vi "Laucher.vi"() -> ()   [LabVIEW 2015]
uses:
  <vilib>/ActorFramework/Actor/Actor.lvclass
panel:
  in  "硬件查询数据间隔":u32=10
  in  "硬件端口":refnum<visa-resource-name>="COM30"
  in  "服务器查询数据间隔":i32=10
  in  "服务器端口":refnum<visa-resource-name>="COM29"
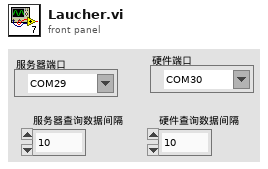
[diagram p1: front panel]
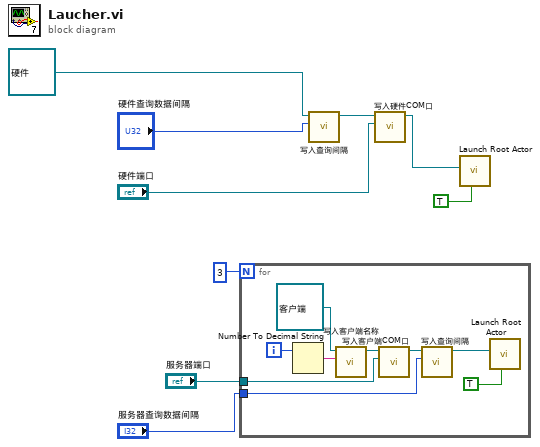
[diagram p0: block diagram]
diagram:
  n1 = for {
    N: 3 -> [_]
    tunnel: "服务器端口" -> [w13]
    tunnel: "服务器查询数据间隔" -> [w12]
    i -> [w17]
    n2 = Number To Decimal String(number=w17) -> (decimal integer string=w16:string)  [unwired: 1 in]
    n3 = call-dynamic "写入客户端名称.vi"("客户端名称"=w16, "客户端输入"=refnum<class "客户端.lvclass"> refnum ("客户端.lvlib:客户端.lvclass")) -> ("客户端输出"=w14:refnum<class "客户端.lvclass">)  [unwired: 8 in, 1 out]
    n4 = call-dynamic "写入客户端COM口.vi"("客户端COM口"=w13, "客户端输入"=w14) -> ("客户端输出"=w11:refnum<class "客户端.lvclass">)  [unwired: 8 in, 1 out]
    n5 = call-dynamic "写入查询间隔.vi"("查询间隔"=w12, "客户端输入"=w11) -> ("客户端输出"=w10:refnum<class "客户端.lvclass">)  [unwired: 8 in, 1 out]
    n6 = call <vilib>:"Launch Root Actor.vi"("Open Actor Core front panel? (F)"=TRUE, "Actor"=w10) -> ()  [unwired: 8 in, 2 out]
  }
  n7 = call-dynamic "写入查询间隔.vi"("查询间隔"="硬件查询数据间隔", "硬件输入"=refnum<class "硬件.lvclass"> refnum ("硬件.lvlib:硬件.lvclass")) -> ("硬件输出"=w4:refnum<class "硬件.lvclass">)  [unwired: 8 in, 1 out]
  n8 = call-dynamic "写入硬件COM口.vi"("硬件COM口"="硬件端口", "硬件输入"=w4) -> ("硬件输出"=w1:refnum<class "硬件.lvclass">)  [unwired: 8 in, 1 out]
  n9 = call <vilib>:"Launch Root Actor.vi"("Open Actor Core front panel? (F)"=TRUE, "Actor"=w1) -> ()  [unwired: 8 in, 2 out]
